vi "Object Detection SubVI experimental.vi"(4 "Error In":errorcluster, 5 "Mode":enum16{"Ball", "Soap", "Gel", "Pipe", "None"}(ring), 6 "Image Dest":T1, 7 "Image in":T1) -> (0 "Error out":errorcluster, 1 "Object Center Coordinates":cluster{"x":sgl, "y":sgl}, 2 "Object detection cluster":T2, 3 "Image Out":T1)   [LabVIEW 2018]
uses:
  <vilib>/vision/Image Controls.llb/IMAQ Image.ctl
panel:
  out "Image":T1(plugin-control)
  out "Ball detected":bool
  out "Pipe detected":bool
  out "Gel detected":bool
  out "Soap detected":bool
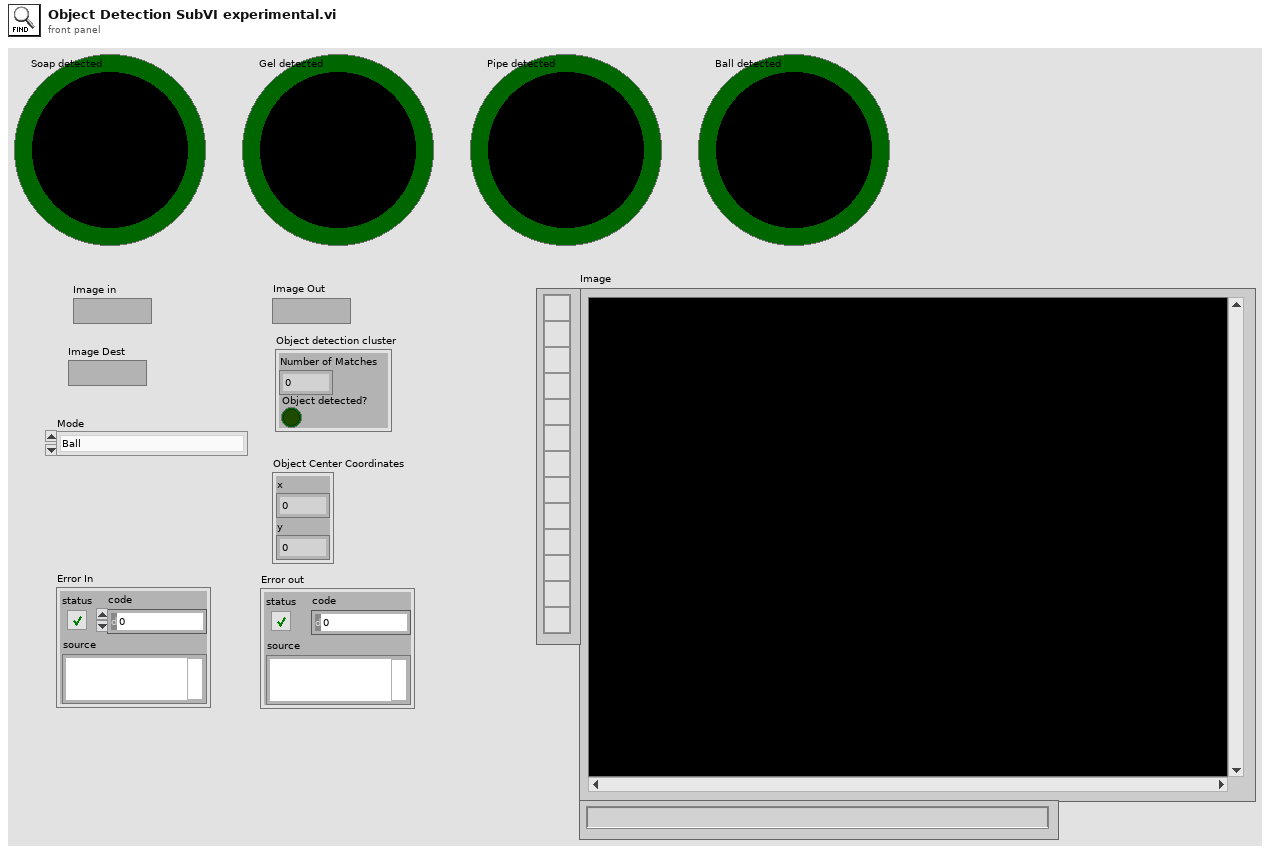
[diagram p1: front panel]
types:
  T1 = typedef "IMAQ Image.ctl" = refnum<image>
  T2 = cluster{"Number of Matches":i32, "Object detected?":bool}
  T3 = cluster{"Position":cluster{"x":sgl, "y":sgl}, "Angle":sgl, "Scale":sgl, "Score":sgl, "Bounding Box":cluster{"x":sgl, "y":sgl}[]}[]
  T4 = typedef "IMAQ GM Match Report.ctl" = cluster{"Position":cluster{"x":sgl, "y":sgl}, "Angle":sgl, "Scale":sgl, "Score":sgl, "Bounding Box":cluster{"x":sgl, "y":sgl}[], "Contrast Reversed":bool, "Occlusion %":sgl, "Template Target Curve Score":sgl, "Target Template Curve Score":sgl, "Correlation Score":sgl}
  T5 = cluster{"Calibrated Matches (Pattern Matching 1)[0]":T4, "Calibrated Matches (Pattern Matching 1)[1]":T4, "Calibrated Matches (Pattern Matching 1)[2]":T4, "Calibrated Matches (Pattern Matching 1)[3]":T4, "Calibrated Matches (Pattern Matching 1)[4]":T4, "Calibrated Matches (Pattern Matching 1)[5]":T4, "Calibrated Matches (Pattern Matching 1)[6]":T4, "Calibrated Matches (Pattern Matching 1)[7]":T4, "Calibrated Matches (Pattern Matching 1)[8]":T4}
  T6 = cluster{"Calibrated Matches (Color Pattern Matching 1)[0]":cluster{"Position":cluster{"x":sgl, "y":sgl}, "Angle":sgl, "Scale":sgl, "Score":sgl, "Bounding Box":cluster{"x":sgl, "y":sgl}[]}, "Calibrated Matches (Color Pattern Matching 1)[1]":cluster{"Position":cluster{"x":sgl, "y":sgl}, "Angle":sgl, "Scale":sgl, "Score":sgl, "Bounding Box":cluster{"x":sgl, "y":sgl}[]}, "Calibrated Matches (Color Pattern Matching 1)[2]":cluster{"Position":cluster{"x":sgl, "y":sgl}, "Angle":sgl, "Scale":sgl, "Score":sgl, "Bounding Box":cluster{"x":sgl, "y":sgl}[]}, "Calibrated Matches (Color Pattern Matching 1)[3]":cluster{"Position":cluster{"x":sgl, "y":sgl}, "Angle":sgl, "Scale":sgl, "Score":sgl, "Bounding Box":cluster{"x":sgl, "y":sgl}[]}, "Calibrated Matches (Color Pattern Matching 1)[4]":cluster{"Position":cluster{"x":sgl, "y":sgl}, "Angle":sgl, "Scale":sgl, "Score":sgl, "Bounding Box":cluster{"x":sgl, "y":sgl}[]}, "Calibrated Matches (Color Pattern Matching 1)[5]":cluster{"Position":cluster{"x":sgl, "y":sgl}, "Angle":sgl, "Scale":sgl, "Score":sgl, "Bounding Box":cluster{"x":sgl, "y":sgl}[]}, "Calibrated Matches (Color Pattern Matching 1)[6]":cluster{"Position":cluster{"x":sgl, "y":sgl}, "Angle":sgl, "Scale":sgl, "Score":sgl, "Bounding Box":cluster{"x":sgl, "y":sgl}[]}, "Calibrated Matches (Color Pattern Matching 1)[7]":cluster{"Position":cluster{"x":sgl, "y":sgl}, "Angle":sgl, "Scale":sgl, "Score":sgl, "Bounding Box":cluster{"x":sgl, "y":sgl}[]}, "Calibrated Matches (Color Pattern Matching 1)[8]":cluster{"Position":cluster{"x":sgl, "y":sgl}, "Angle":sgl, "Scale":sgl, "Score":sgl, "Bounding Box":cluster{"x":sgl, "y":sgl}[]}}
  T7 = cluster{"Position":cluster{"x":sgl, "y":sgl}, "Angle":sgl, "Scale":sgl, "Score":sgl, "Bounding Box":cluster{"x":sgl, "y":sgl}[]}
  T8 = cluster{"Number of Matches (Pattern Matching 1)":i32, bool}
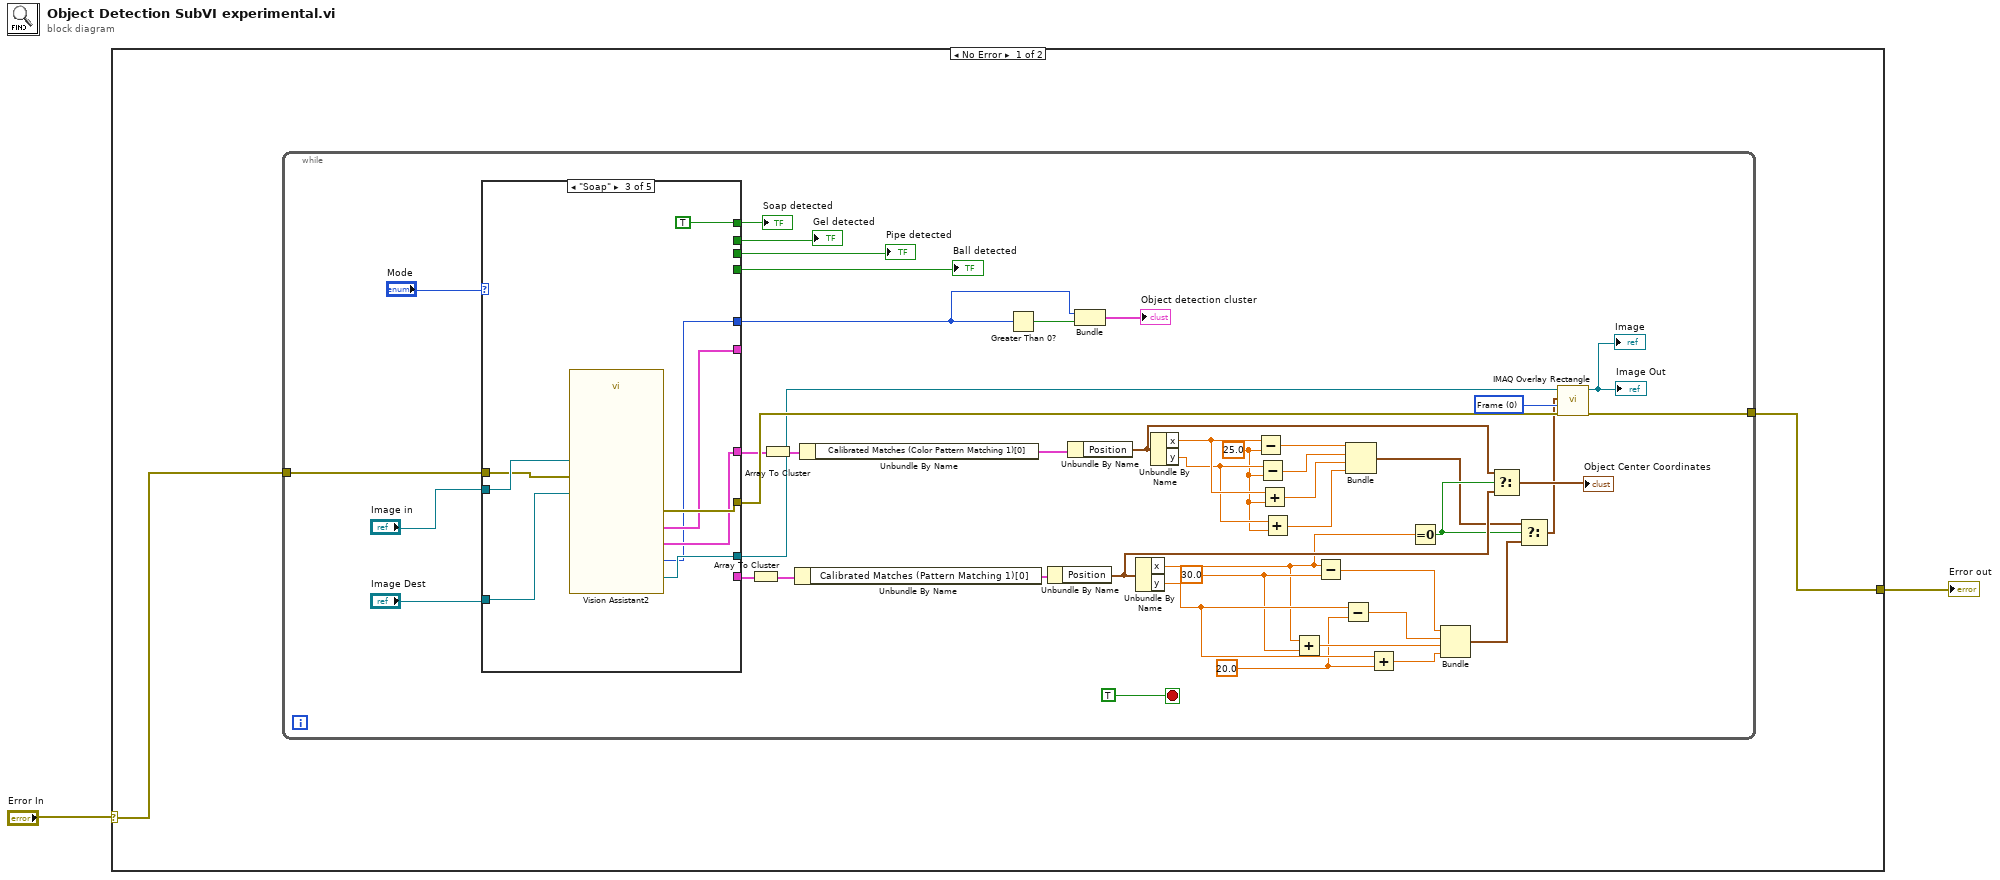
[diagram p0: block diagram]
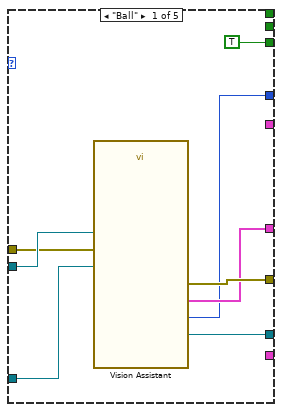
[diagram p2: hidden frame]
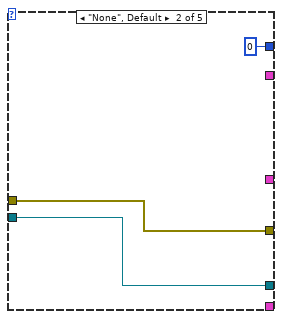
[diagram p3: hidden frame]
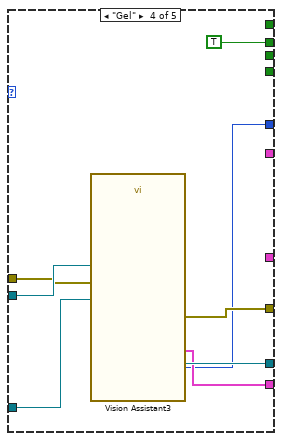
[diagram p4: hidden frame]
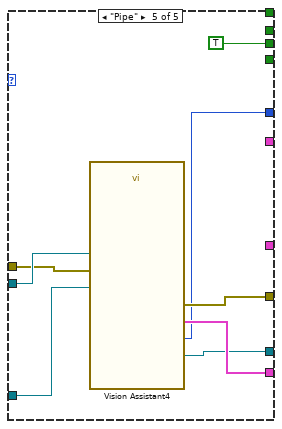
[diagram p5: hidden frame]
diagram:
  n1 = case shown="No Error" "Error In" {
    selector: "Error In" -> [w4 w86]
    tunnel: [w3 w86] -> w2
    frame No Error {
      n2 = while {
        tunnel: w4 -> [w33]
        tunnel: [w32] -> w3
        stop <- TRUE ("Stop (F)") stop-if-true
        w22 = sgl 25.0 ("y")
        w34 = sgl 30.0 ("y")
        w37 = sgl 20.0 ("y")
        w47 = u32 0 items=["Frame", "Fill", "Highlight"] ("Drawing Mode (Frame)")
        n3 = case shown="\"Soap\"" "Mode" {
          tunnel: [w57 w60 w69 w77 w85] -> w46
          tunnel: "Image in" -> [w56 w59 w68 w76 w84]
          tunnel: "Image Dest" -> [w55 _ w67 w75 w83]
          tunnel: [_ _ w66 _ _] -> _
          tunnel: [_ _ _ w71 w82] -> w45
          tunnel: [w54 w59 w65 w74 w81] -> w35
          tunnel: w33 -> [w53 w60 w64 w73 w80]
          tunnel: [_ _ TRUE _ _] -> w31
          tunnel: [_ _ _ TRUE _] -> w30
          tunnel: [_ _ _ _ TRUE] -> w29
          tunnel: [TRUE _ _ _ _] -> w28
          tunnel: [w51 _ w62 _ _] -> w11
          tunnel: [w50 0 ("Number of Matches (Color Pattern Matching 1)") w61 w70 w78] -> w6
          frame "Ball" {
            n4 = call "Vision Assistant"("Image In"=w56, "Image Dst"=w55, "error in"=w53) -> ("Image Out"=w54:T1, "Number of Matches (Color Location 1)"=w50:i32, "Matches (calibrated) (Color Location 1)"=w51:T3, "error out"=w57:errorcluster)  [unwired: 20 in, 1 out]
          }
          frame "None", Default {
          }
          frame "Soap" {
            n5 = call "Vision Assistant2"("Image In"=w68, "Image Dst"=w67, "error in"=w64) -> ("Image Out"=w65:T1, "Matches (Color Pattern Matching 1)"=w66:T3, "Calibrated Matches (Color Pattern Matching 1)"=w62:T3, "Number of Matches (Color Pattern Matching 1)"=w61:i32, "error out"=w69:errorcluster)  [unwired: 20 in]
          }
          frame "Gel" {
            n6 = call "Vision Assistant3"("Image In"=w76, "Image Dst"=w75, "error in"=w73) -> ("Image Out"=w74:T1, "Calibrated Matches (Pattern Matching 1)"=w71:T4[], "Number of Matches (Pattern Matching 1)"=w70:i32, "error out"=w77:errorcluster)  [unwired: 20 in, 1 out]
          }
          frame "Pipe" {
            n7 = call "Vision Assistant4"("Image In"=w84, "Image Dst"=w83, "error in"=w80) -> ("Image Out"=w81:T1, "Number of Matches (Pattern Matching 1)"=w78:i32, "Calibrated Matches (Pattern Matching 1)"=w82:T4[], "error out"=w85:errorcluster)  [unwired: 20 in, 1 out]
          }
        }
        "Soap detected" <- w31
        "Pipe detected" <- w29
        "Ball detected" <- w28
        "Gel detected" <- w30
        n8 = Array To Cluster(array=w45) -> (cluster=w44:T5)
        n9 = Array To Cluster(array=w11) -> (cluster=w10:T6)
        n10 = Unbundle By Name(w44) -> ("Calibrated Matches (Pattern Matching 1)[0]"=w43:T4)
        n11 = Unbundle By Name(w10) -> ("Calibrated Matches (Color Pattern Matching 1)[0]"=w9:T7)
        n12 = Greater Than 0?(x=w6) -> (x > 0?=w7:bool)
        n13 = Unbundle By Name(w43) -> ("Position"=w18:cluster{"x":sgl, "y":sgl})
        n14 = Unbundle By Name(w9) -> ("Position"=w17:cluster{"x":sgl, "y":sgl})
        n15 = Bundle("Number of Matches (Pattern Matching 1)"=w6, w7) -> (→"Object detection cluster":T8)  [unwired: 1 in]
        n16 = Unbundle By Name(w18) -> ("x"=w16:sgl, "y"=w39:sgl)
        n17 = Unbundle By Name(w17) -> ("x"=w24:sgl, "y"=w23:sgl)
        n18 = Subtract(x=w24, y=w22) -> (x-y=w26:sgl)
        n19 = Subtract(x=w23, y=w22) -> (x-y=w25:sgl)
        n20 = Add(x=w24, y=w22) -> (x+y=w21:sgl)
        n21 = Add(x=w23, y=w22) -> (x+y=w20:sgl)
        n22 = Add(x=w16, y=w34) -> (x+y=w42:sgl)
        n23 = Subtract(x=w16, y=w34) -> (x-y=w40:sgl)
        n24 = Subtract(x=w39, y=w37) -> (x-y=w38:sgl)
        n25 = Bundle(w26, w25, w21, w20) -> (w13:cluster{sgl, sgl, sgl, sgl})  [unwired: 1 in]
        n26 = Add(x=w39, y=w37) -> (x+y=w41:sgl)
        n27 = Equal To 0?(x=w16) -> (x = 0?=w14:bool)
        n28 = Bundle(w40, w38, w42, w41) -> (w15:cluster{sgl, sgl, sgl, sgl})  [unwired: 1 in]
        n29 = Select(t=w17, s=w14, f=w18) -> (s? t:f=→"Object Center Coordinates":cluster{"x":sgl, "y":sgl})
        n30 = Select(t=w13, s=w14, f=w15) -> (s? t:f=w12:cluster{sgl, sgl, sgl, sgl})
        n31 = call "IMAQ Overlay Rectangle"("error in (no error)"=w46, "Drawing Mode (Frame)"=w47, "Rectangle"=w12, "Image"=w35) -> ("error out"=w32:errorcluster, "Image Out"=→"Image Out" →"Image":T1)  [unwired: 6 in]
      }
    }
    frame Error {
    }
  }
  "Error out" <- w2
